vi "dll.midi_destroy_manager.vi"(8 "error in (no error)":errorcluster, 11 "midi out in":refnum<class "midi out.lvclass">) -> (0 "error out":errorcluster, 3 "midi out out":refnum<class "midi out.lvclass">)   [LabVIEW 2020, in "midi out.lvclass"]
uses:
  midi out.lvclass
  midi out.lvclass/midi out.ctl
  shared/midi shared.lvlib
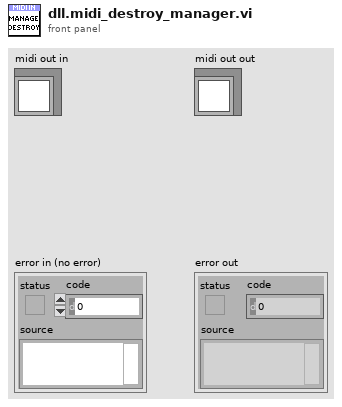
[diagram p1: front panel]
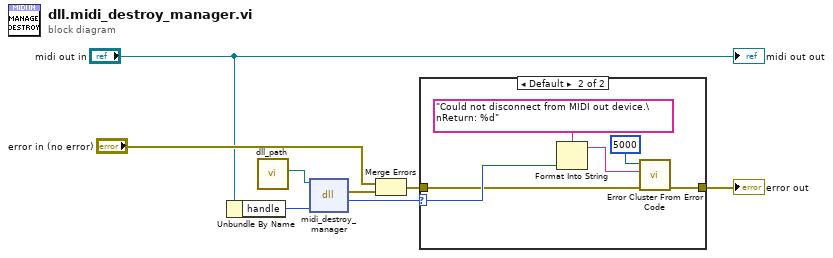
[diagram p0: block diagram]
diagram:
  n1 = Unbundle By Name("midi out in") -> ("handle"=w6:i32)
  n2 = call "dll_path.vi"() -> ("dll"=w8:path)  [unwired: 11 in]
  n3 = dll-call lib="C:/code/LabVIEW-MIDI-XPLAT/dist/TomMIDIllan_*.*" fn="midi_destroy_manager"(path in=w8, "handle"=w6) -> (error out=w4:errorcluster, "return"=w5:i32)  [unwired: 3 in, 1 out]
  n4 = Merge Errors("error in (no error)", w4) -> (w7:errorcluster)
  n5 = case shown="Default" w5 {
    selector: w5 -> [_ w12]
    tunnel: w7 -> [w9 w11]
    tunnel: [w9 w10] -> w1
    frame 0.. {
    }
    frame Default {
      n6 = Format Into String(format string="Could not disconnect from MIDI out device.\nReturn: %d", w12) -> (resulting string=w13:string)  [unwired: 2 in, 1 out]
      n7 = call <vilib>:"Error Cluster From Error Code.vi"("error in (no error)"=w11, "error message (\"\")"=w13, "error code (0)"=5000) -> ("error out"=w10:errorcluster)  [unwired: 6 in]
    }
  }
  "error out" <- w1
  "midi out out" <- "midi out in"
